vi "ANSIfloat.vi"() -> ()   [LabVIEW 2023]
doc: "This function squares the value of input and returns the value in output.\n\nFor information on the data types used for the DLL function, right-click on the Call Library Function node and choose Configure."
uses:
  CLF_Example.dll
panel:
  out "output":sgl format="%0.2f"
  in  "input":sgl=10.0 format="%0.2f"
  # "See the block diagram for more information."
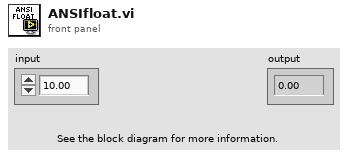
[diagram p1: front panel]
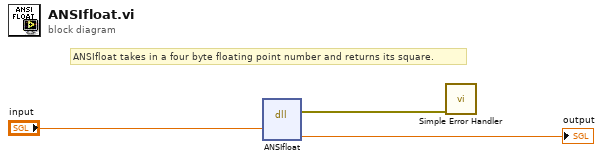
[diagram p0: block diagram]
diagram:
  # "ANSIfloat takes in a four byte floating point number and returns its square."
  n1 = dll-call lib="c:/dev/_r/4/eng/lv-core/lvpostprocessingd/lv_mc_x86_64/dist_i386/examples/Connectivity/Libraries and Executables/DLL Calling VIs/CLF_Example**.*" fn="ANSIfloat"("input"="input") -> (error out=w1:errorcluster, "output"=→"output":sgl)  [unwired: 4 in, 3 out]
  n2 = call <vilib>:"Simple Error Handler.vi"("error in (no error)"=w1) -> ()  [unwired: 4 in, 5 out]
